vi "Run Service.vi"() -> ()   [LabVIEW 2021, in "dcvmDPI_AD7606B_server.lvlib"]
uses:
  dcvmDPI_AD7606B_server.lvlib
  RPC Service/dcvmDPI/dcvmDPI.lvclass
  C:/Program Files/National Instruments/LabVIEW 2021/vi.lib/gRPC/LabVIEW gRPC Servicer/ServiceBase/ServiceBase.lvclass
  <vilib>/gRPC/LabVIEW gRPC Servicer/Servicer/Servicer.lvclass/Servicer.ctl
  <vilib>/gRPC/LabVIEW gRPC Servicer/Servicer/Servicer.lvclass
  dcvmMessageQueue/dcvmMessageQueue.lvlib
  dcvmDPI_AD7606B_serverImpl/dcvmDPI_AD7606B_serverImpl.lvlib
panel:
  out "Listening Port":i32
  in  "Stop":bool
  in  "Server Address":string="localhost:50051"
  in  "Server Certificate File (.crt)":path
  in  "Server Key File (.key)":path
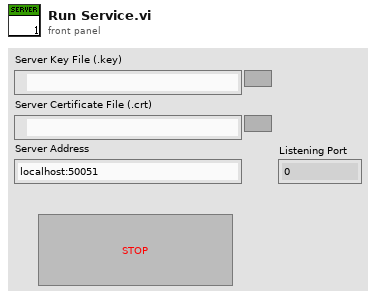
[diagram p1: front panel]
types:
  T1 = typedef "grpc-lvsupport-release.lvlib/grpcId.ctl" = u64
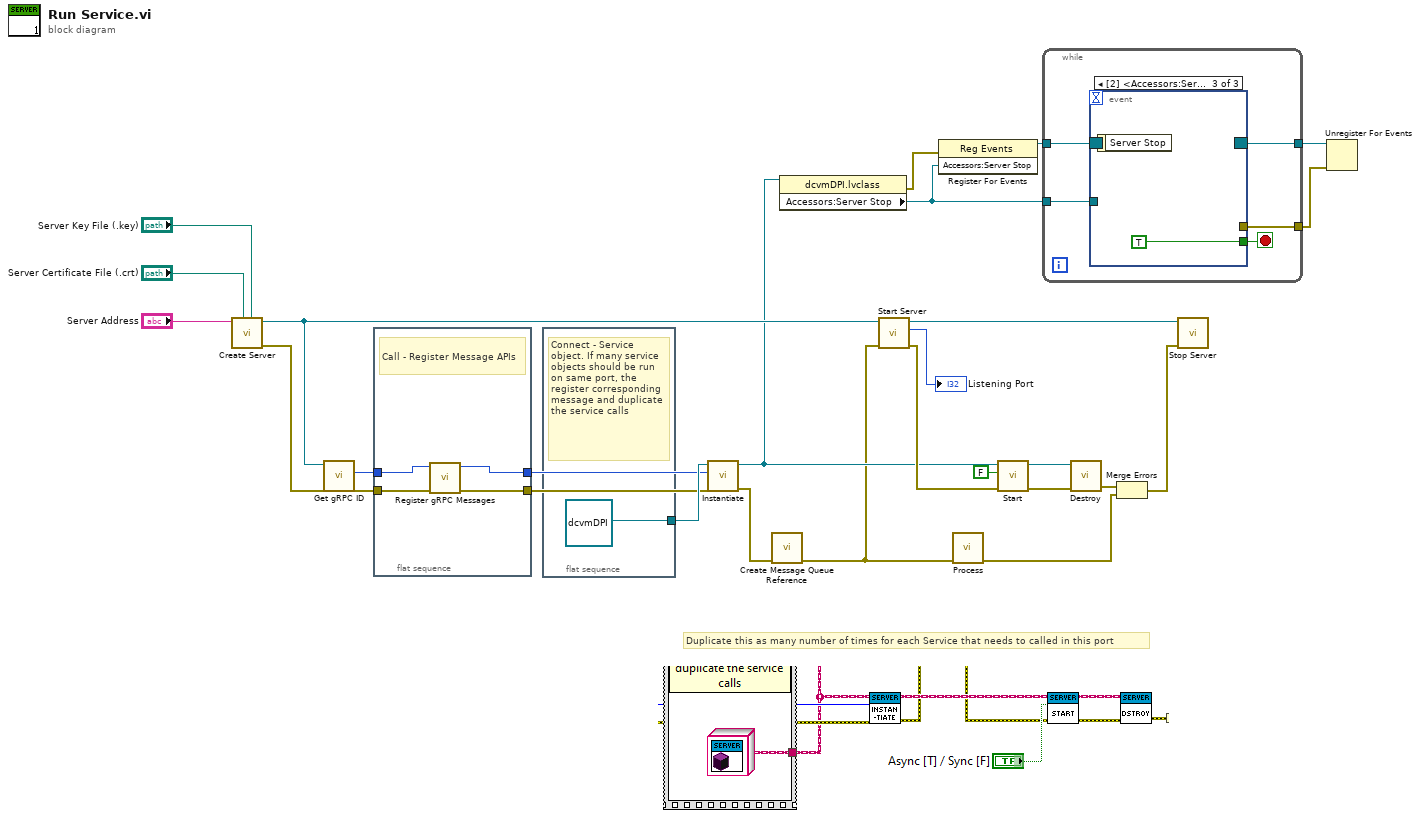
[diagram p0: block diagram]
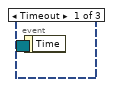
[diagram p2: hidden frame]
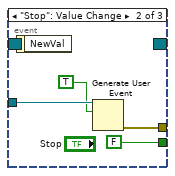
[diagram p3: hidden frame]
diagram:
  # "Duplicate this as many number of times for each Service that needs to called in this port"
  n1 = call <vilib>:"Create Server.vi"("Server Key File (.key)"="Server Key File (.key)", "Server Certificate File (.crt)"="Server Certificate File (.crt)", "Server Address"="Server Address") -> ("error out"=w12:errorcluster, "gRPC Server out"=w19:refnum<class "Servicer.lvclass">)  [unwired: 7 in]
  n2 = call <vilib>:"Get gRPC ID.vi"("OOP Server in"=w19) -> ("gRPC ID"=w13:T1)  [unwired: 9 in, 1 out]
  n3 = flat-sequence {
    tunnel: w13 -> [w28]
    tunnel: w12 -> [w30]
    tunnel: [w29] -> w11
    tunnel: [w27] -> w10
    frame #0 {
      # "Call - Register Message APIs"
      n4 = call "Register gRPC Messages.vi"("error in (no error)"=w30, "gRPC ID"=w28) -> ("error out"=w29:errorcluster, "gRPC ID Out"=w27:T1)  [unwired: 8 in]
    }
  }
  n5 = flat-sequence {
    tunnel: [refnum<class "dcvmDPI.lvclass"> refnum ("dcvmDPI_AD7606B_server.lvlib:dcvmDPI.lvclass")] -> w14
    frame #0 {
      # "Connect - Service object. If many service objects should be run on same port, the register corresponding message and duplicate the service calls"
    }
  }
  n6 = call-dynamic "Instantiate.vi"("error in"=w11, "gRPCid"=w10, "iService"=w14) -> ("error out"=w3:errorcluster, "iService"=w6:refnum<class "dcvmDPI.lvclass">)  [unwired: 7 in]
  n7 = call "Create Message Queue Reference.vi"("error in (no error)"=w3) -> ("error out"=w2:errorcluster)  [unwired: 10 in]
  n8 = property class="dcvmDPI.lvclass"(reference=w6) -> (error out=w18:errorcluster, "Accessors:Server Stop"=w5:refnum<user-event>)  [unwired: 1 in, 1 out]
  n9 = call <vilib>:"Start Server.vi"("error in"=w2, "gRPC Server in"=w19) -> ("error out"=w9:errorcluster, "Listening Port"=→"Listening Port":i32, "gRPC Server out"=w26:refnum<class "Servicer.lvclass">)  [unwired: 7 in]
  n10 = register-events(error in=w18, w5) -> (reference out=w22:refnum<event-registration>)  [unwired: 1 in, 1 out]
  n11 = call "Process.vi"("error in"=w2) -> ("error out"=w1:errorcluster)  [unwired: 10 in]
  n12 = call-dynamic "Start.vi"("error in"=w9, "ASync [T]"=FALSE, "iService in"=w6) -> ("error out"=w8:errorcluster, "iService out"=w7:refnum<class "dcvmDPI.lvclass">)  [unwired: 7 in]
  n13 = while {
    tunnel: w22 -> [w36]
    tunnel: [w34] -> w21
    tunnel: [w32] -> w15
    tunnel: w5 -> [w33]
    stop <- w35 stop-if-true
    n14 = event shown="[2] <Accessors:Server Stop>: User Event" {
      selector: w36 -> [_ _ _]
      dyn-events: [_ _ _] -> w34
      timeout: _ -> [_ _ _]
      tunnel: [_ FALSE TRUE] -> w35
      tunnel: w33 -> [_ w39 _]
      tunnel: [_ w37 _] -> w32
      event Timeout {
        n15 = event-data() -> ()  [unwired: 1 in, 1 out]
      }
      event "Stop": Value Change {
        n16 = event-data() -> ()  [unwired: 1 in, 1 out]
        n17 = Generate User Event(user event=w39, event data cluster=TRUE ("event data")) -> (error out=w37:errorcluster)  [unwired: 2 in, 1 out]
      }
      event User Event {
        n18 = event-data() -> ()  [unwired: 1 in, 1 out]
      }
    }
  }
  n19 = call-dynamic "Destroy.vi"("error in (no error)"=w8, "SignalGeneratorService in"=w7) -> ("error out"=w17:errorcluster)  [unwired: 8 in, 1 out]
  n20 = Merge Errors(w17, w1) -> (w16:errorcluster)
  n21 = call <vilib>:"Stop Server.vi"("error in"=w16, "gRPC Server in"=w26) -> ()  [unwired: 9 in, 1 out]
  n22 = Unregister For Events(event registration refnum=w21, error in=w15) -> ()  [unwired: 1 out]
